vi "Fetch&Process_Measurements_V2.vi"(7 "Rolling Timer Input Array":timestamp[](array[timestamp]), 8 "error in":errorcluster, 10 "Initial Time Array":timestamp[](array[timestamp]), 11 "DCPowerInformation_byChannel":T2(array[cluster])) -> (0 "error output":errorcluster, 1 "Current Measurements":waveform(dbl)[](array[waveform]), 2 "Voltage Measurements":waveform(dbl)[](array[waveform]), 3 "Queue Data Parameters output":T1, 5 "Rolling Time Output Array":timestamp[](array[timestamp]))   [LabVIEW 2019]
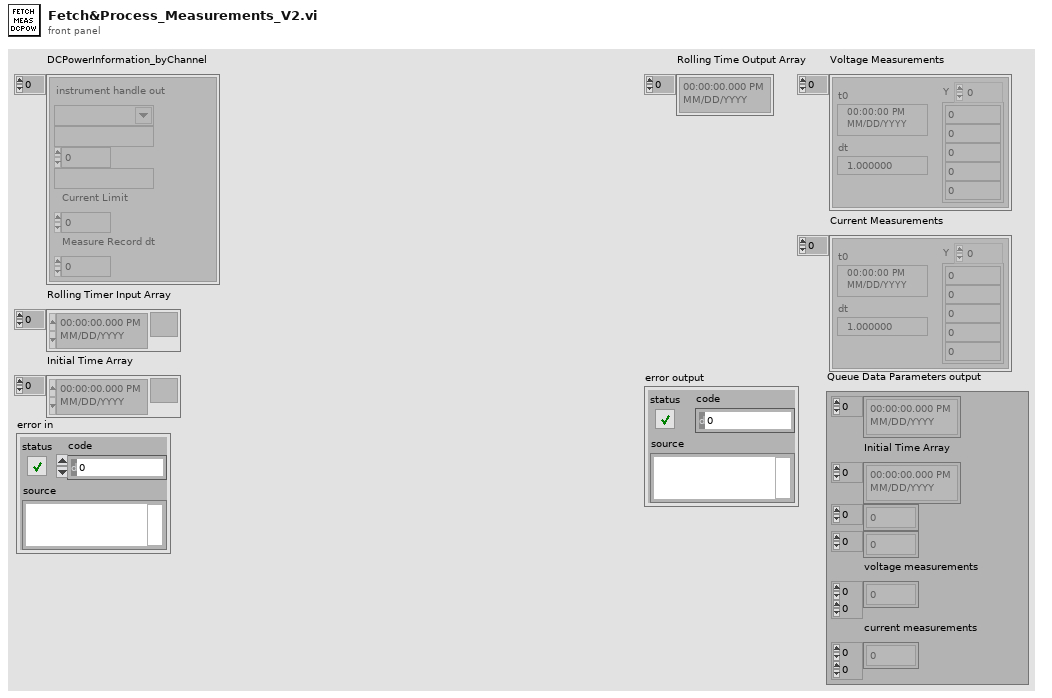
[diagram p1: front panel]
types:
  T1 = cluster{timestamp[], "Initial Time Array":timestamp[], i32[], dbl[], "voltage measurements":dbl[][], "current measurements":dbl[][]}
  T2 = cluster{"instrument handle out":refnum<k15>, string, dbl, string, "Current Limit":dbl, "Measure Record dt":dbl}[]
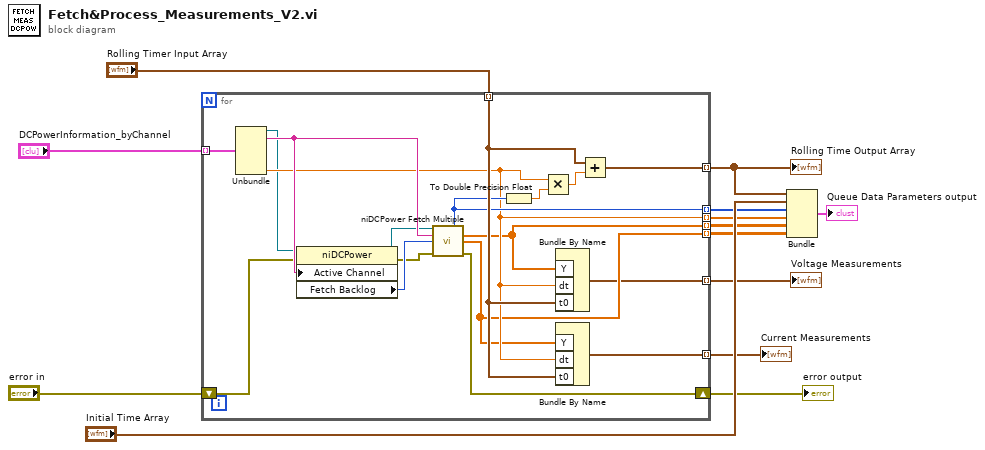
[diagram p0: block diagram]
diagram:
  n1 = for {
    tunnel: "DCPowerInformation_byChannel" -> [w31] mode=indexing
    shift-right: [w28] -> w1
    shift-left: "error in" -> [w16]
    tunnel: "Rolling Timer Input Array" -> [w24] mode=indexing
    tunnel: [w25] -> w10 mode=indexing
    tunnel: [w23] -> w8 mode=indexing
    tunnel: [w22] -> w7 mode=indexing
    tunnel: [w21] -> w6 mode=indexing
    tunnel: [w20] -> w5 mode=indexing
    tunnel: [w19] -> w4 mode=indexing
    tunnel: [w18] -> w3 mode=indexing
    n2 = Unbundle(w31) -> ("instrument handle out"=w17:refnum<k15>, w30:string, "Measure Record dt"=w22:dbl)  [unwired: 3 out]
    n3 = property class="niDCPower"(reference=w17, error in=w16, "Active Channel"=w30) -> (reference out=w14:refnum<k15>, error out=w15:errorcluster, "Fetch Backlog"=w29:i32)
    n4 = call <instrlib>:"niDCPower Fetch Multiple.vi"("instrument handle"=w14, "channel name"=w30, "count (1)"=w29, "error in (no error)"=w15) -> ("actual count"=w23:i32, "voltage measurements"=w21:dbl[], "current measurements"=w20:dbl[], "error out"=w28:errorcluster)  [unwired: 6 in, 2 out]
    n5 = To Double Precision Float(number=w23) -> (double precision float=w27:dbl)
    n6 = Multiply(x=w22, y=w27) -> (x*y=w26:dbl)
    n7 = Bundle By Name("Y"=w21, "dt"=w22, "t0"=w24) -> (w19:waveform(dbl))  [unwired: 1 out]
    n8 = Bundle By Name("Y"=w20, "dt"=w22, "t0"=w24) -> (w18:waveform(dbl))  [unwired: 1 out]
    n9 = Add(x=w24, y=w26) -> (x+y=w25:timestamp)
  }
  "Voltage Measurements" <- w4
  "Current Measurements" <- w3
  "Rolling Time Output Array" <- w10
  "error output" <- w1
  n10 = Bundle(w10, "Initial Time Array"="Initial Time Array", w8, w7, "voltage measurements"=w6, "current measurements"=w5) -> (→"Queue Data Parameters output":T1)  [unwired: 1 in]
